vi "ConvertBlob.vi"(11 "Measurements":dbl[](array[numeric])) -> (3 "Converted Blob":T1 {"Equiv. Rect"."Height" format="%.2f"; "Equiv. Rect"."Width" format="%.2f"; "Center of Mass"."Y" format="%.2f"; "Center of Mass"."X" format="%.2f"; "Bounding Rect"."Bottom" format="%.2f"; "Bounding Rect"."Right" format="%.2f"; "Bounding Rect"."Top" format="%.2f"; "Bounding Rect"."Left" format="%.2f"; "Area" format="%.2f"})   [LabVIEW 2013]
uses:
  BlobMeasurementType.ctl
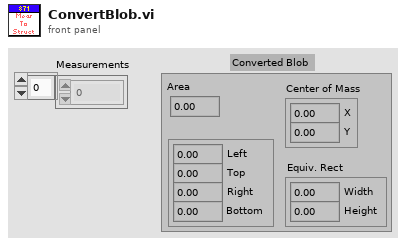
[diagram p1: front panel]
types:
  T1 = typedef "BlobMeasurementType.ctl" = cluster{"Area":dbl, "Bounding Rect":cluster{"Left":dbl, "Top":dbl, "Right":dbl, "Bottom":dbl}, "Center of Mass":cluster{"X":dbl, "Y":dbl}, "Equiv. Rect":cluster{"Width":dbl, "Height":dbl}}
  T2 = cluster{"Numeric":dbl, "Numeric":dbl, "Numeric":dbl, "Numeric":dbl}
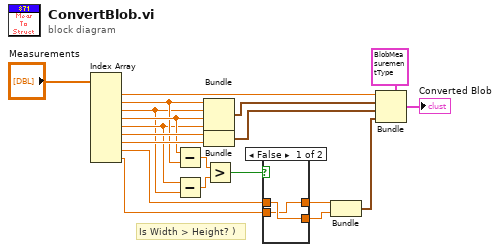
[diagram p0: block diagram]
diagram:
  # "Is Width > Height? )"
  n1 = Index Array(array="Measurements") -> (element #1=w19:dbl, element #2=w11:dbl, element #3=w9:dbl, element #4=w12:dbl, element #5=w10:dbl, element #6=w15:dbl, element #7=w14:dbl, element #8=w5:dbl, element #9=w4:dbl)  [unwired: 9 in]
  n2 = Subtract(x=w12, y=w11) -> (x-y=w8:dbl)
  n3 = Subtract(x=w10, y=w9) -> (x-y=w7:dbl)
  n4 = Bundle("Numeric"=w11, "Numeric"=w9, "Numeric"=w12, "Numeric"=w10) -> (w16:T2)  [unwired: 1 in]
  n5 = Bundle("Numeric"=w15, "Numeric"=w14) -> (w13:cluster{"Numeric":dbl, "Numeric":dbl})  [unwired: 1 in]
  n6 = Greater?(x=w8, y=w7) -> (0:w6:bool)
  n7 = case shown="False" w6 {
    tunnel: w5 -> [w22 w24]
    tunnel: w4 -> [w21 w23]
    tunnel: [w21 w24] -> w2
    tunnel: [w22 w23] -> w1
    frame False {
    }
    frame True {
    }
  }
  n8 = Bundle("Numeric"=w2, "Numeric"=w1) -> (w3:cluster{"Numeric":dbl, "Numeric":dbl})  [unwired: 1 in]
  n9 = Bundle(cluster=T1 {"Area"=0.0, "Bounding Rect"={"Left"=0.0, "Top"=0.0, "Right"=0.0, "Bottom"=0.0}, "Center of Mass"={"X"=0.0, "Y"=0.0}, "Equiv. Rect"={"Width"=0.0, "Height"=0.0}} ("Particle Report"), "Area"=w19, "Bounding Rect"=w16, "Center of Mass"=w13, "Equiv. Rect"=w3) -> (→"Converted Blob":T1)
